vi "stage_get_position.vi"(8 "error in (no error)":errorcluster, 10 "Stage Name":string, 11 "Stage in":refnum<class "thorlabs_kinesis.lvclass">) -> (0 "error out":errorcluster, 2 "Position":dbl, 3 "Stage out":refnum<class "thorlabs_kinesis.lvclass">)   [LabVIEW 2015, in "thorlabs_kinesis.lvclass"]
uses:
  thorlabs_kinesis.lvclass
  thorlabs_kinesis.lvclass/thorlabs_kinesis.ctl
  thorlabs_drivers/Thorlabs.MotionControl.Benchtop.Piezo.dll
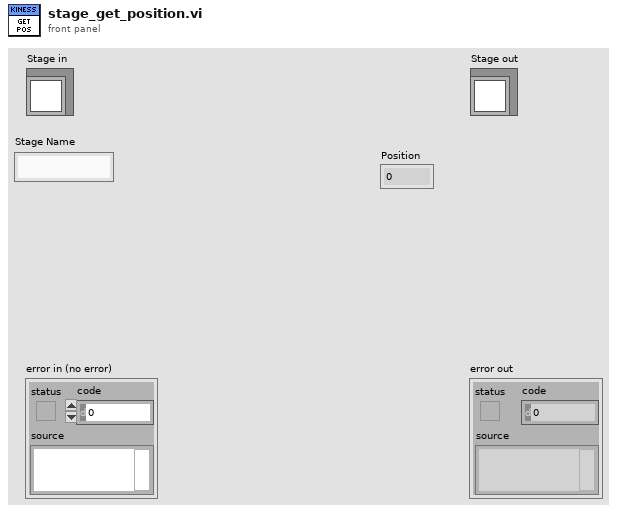
[diagram p1: front panel]
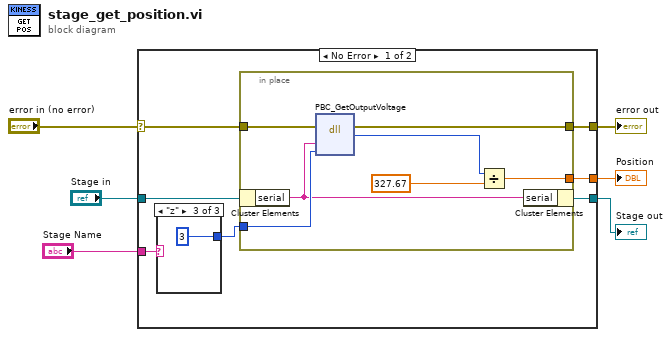
[diagram p0: block diagram]
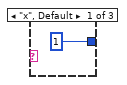
[diagram p2: hidden frame]
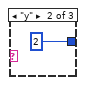
[diagram p3: hidden frame]
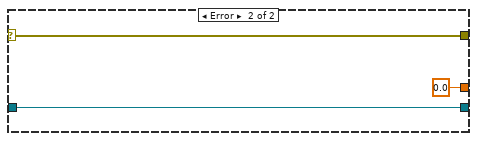
[diagram p4: hidden frame]
diagram:
  n1 = case shown="No Error" "error in (no error)" {
    selector: "error in (no error)" -> [w9 w26]
    tunnel: [w8 w26] -> w5
    tunnel: [w10 w25] -> w3
    tunnel: "Stage in" -> [w11 w25]
    tunnel: "Stage Name" -> [w13 _]
    tunnel: [w7 0.0] -> w1
    frame No Error {
      n2 = case shown="\"z\"" w13 {
        tunnel: [i16 1 ("channel") i16 2 ("channel") i16 3 ("channel")] -> w12
        frame "x", Default {
        }
        frame "y" {
        }
        frame "z" {
        }
      }
      n3 = in-place {
        in-place-border: w9 -> [w23]
        in-place-border: w12 -> [w22]
        in-place-border: [w20] -> w8
        in-place-border: [w17] -> w7
        n4 = in-place-cluster #1(w11) -> ("serial"=w21:string)
        n5 = dll-call lib="C:/Users/bspoka/Documents/LabVIEW Data/lview_180307/Stage Class/Thorlabs Kinesis/thorlabs_drivers/Thorlabs.MotionControl.Benchtop.Piezo.dll" fn="PBC_GetOutputVoltage"(error in=w23, "serial"=w21, "channel"=w22) -> (error out=w20:errorcluster, "return type"=w19:i16)  [unwired: 4 in, 1 out]
        n6 = Divide(x=w19, y=327.67) -> (x/y=w17:dbl)
        n7 = in-place-cluster #1("serial"=w21) -> (w10:refnum<class "thorlabs_kinesis.lvclass">)
      }
    }
    frame Error {
    }
  }
  "error out" <- w5
  "Stage out" <- w3
  "Position" <- w1
